vi "mock test.vi"() -> ()   [LabVIEW 2020]
panel:
  out "Array 2":i32[](array[numeric])
  out "appended array":dbl[][](array[numeric])
  out "Array":dbl[](array[numeric])
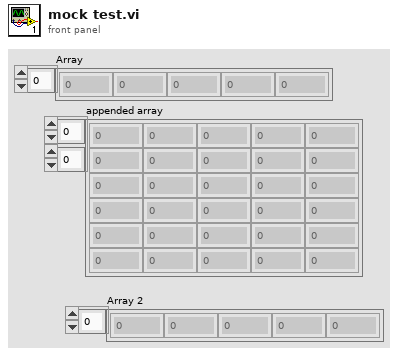
[diagram p1: front panel]
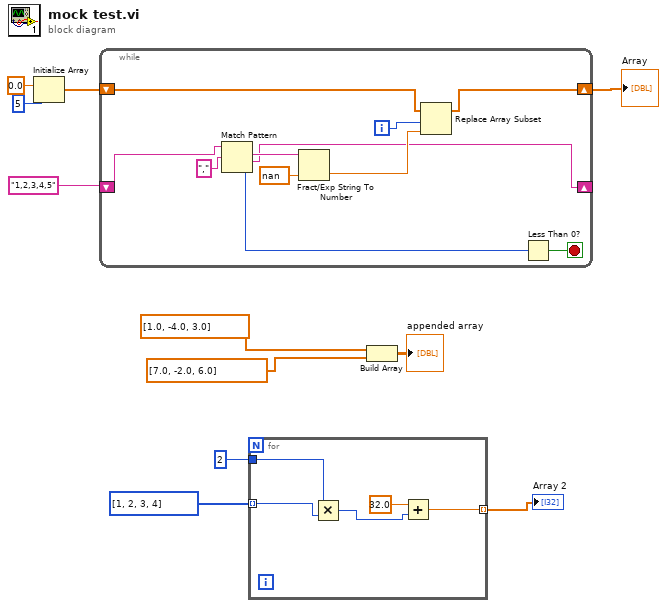
[diagram p0: block diagram]
diagram:
  n1 = Initialize Array(0.0 ("element"), 5 ("dimension size")) -> (w8:dbl[])
  n2 = while {
    shift-right: [w21] -> w7
    shift-left: w8 -> [w22]
    shift-right: [w12] -> _
    shift-left: "1,2,3,4,5" -> [w19]
    i -> [w20]
    stop <- w13 stop-if-true
    n3 = Match Pattern(string=w19, regular expression=",") -> (before substring=w17:string, after substring=w12:string, offset past match=w14:i32)  [unwired: 1 in, 1 out]
    n4 = Fract/Exp String To Number(string=w17, default (0 dbl)=nan ("default (0 DBL)")) -> (number=w15:dbl)  [unwired: 2 in, 1 out]
    n5 = Replace Array Subset(array=w22, new element=w15, index=w20) -> (w21:dbl[])
    n6 = Less Than 0?(x=w14) -> (x < 0?=w13:bool)
  }
  "Array" <- w7
  n7 = for {
    tunnel: i32[] [1, 2, 3, 4] -> [w25] mode=indexing
    tunnel: 2 -> [w24]
    tunnel: [w23] -> w1 mode=indexing
    n8 = Multiply(x=w24, y=w25) -> (x*y=w26:i32)
    n9 = Add(x=32.0, y=w26) -> (x+y=w23:dbl)
  }
  "Array 2" <- w1
  n10 = Build Array(dbl[] [1.0, -4.0, 3.0], dbl[] [7.0, -2.0, 6.0]) -> (→"appended array":dbl[][])
